vi "PR_error_spout .vi"(7 "[workplace_id]":i16=2, 8 "error in (no error)":errorcluster, 9 "QC result":string="NG,", 10 "barcode":string="123465798", 11 "DBlink":string="Driver={ODBC Driver 17 for SQL Server};Server=localhost\\SQLEXPRESS;Database=ZDX201;UID=labview;PWD=Dsa@54137926") -> (0 "error out":errorcluster)   [LabVIEW 2019]
uses:
  <vilib>/addons/database/Connection.llb/DB Tools Open Connec (String).vi
  <vilib>/addons/database/NI_Database_API.lvlib
panel:
  out "concatenated string":string="WHERE [barcode]='123465798' and [pos]='A'"
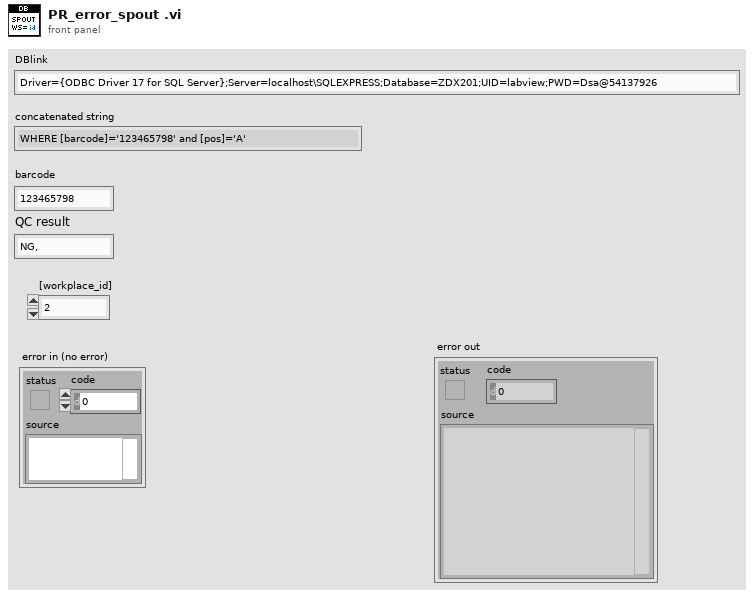
[diagram p1: front panel]
types:
  T1 = cluster{"[workplace_id]":i16, "[time_spout]":timestamp, "QC result":string}
  T2 = typedef "NI_Database_API.lvlib/Conn ObjectReference.ctl" = refnum<k1>
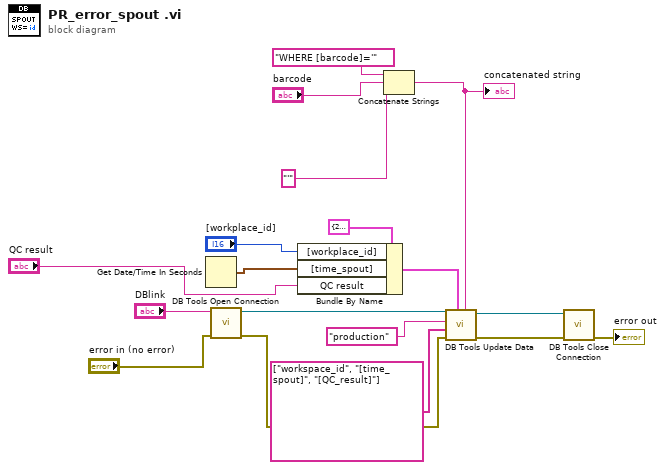
[diagram p0: block diagram]
diagram:
  n1 = Get Date/Time In Seconds() -> (seconds since 1Jan1904=w3:timestamp)
  n2 = call-poly <vilib>:"DB Tools Open Connection.vi"("error in (no error)"="error in (no error)", "connection information"="DBlink") -> ("error out"=w16:errorcluster, "connection reference"=w14:T2)  [unwired: 6 in]
  n3 = Bundle By Name(cluster=T1 {"[workplace_id]"=2, "[time_spout]"=timestamp(0 s since 1904-01-01), "QC result"="'"}, "[workplace_id]"="[workplace_id]", "[time_spout]"=w3, "QC result"="QC result") -> (w2:T1)
  n4 = Concatenate Strings("WHERE [barcode]='", "barcode", "'" ("string")) -> (w8:string)
  "concatenated string" <- w8
  n5 = call <vilib>:"DB Tools Update Data.vi"("condition"=w8, "data"=w2, "error in (no error)"=w16, "columns"=string[] ["workspace_id", "[time_spout]", "[QC_result]"], "table"="production", "connection reference"=w14) -> ("error out"=w17:errorcluster, "connection reference out"=w15:T2)  [unwired: 4 in]
  n6 = call <vilib>:"DB Tools Close Connection.vi"("error in (no error)"=w17, "connection reference"=w15) -> ("error out"=→"error out":errorcluster)  [unwired: 5 in]
